vi "errorToString.vi"(1 "error in":errorcluster) -> (0 "Error Message":string)   [LabVIEW 2021]
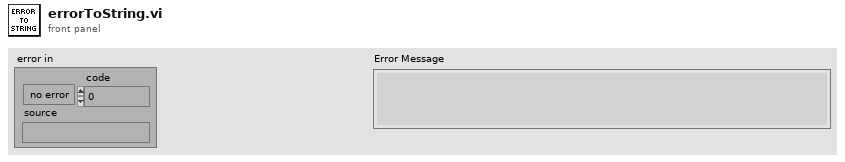
[diagram p1: front panel]
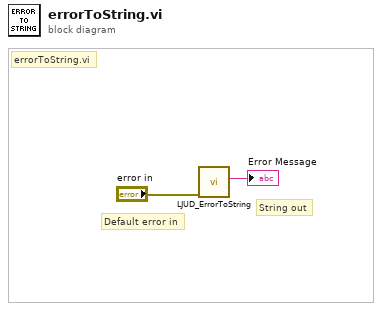
[diagram p0: block diagram]
diagram:
  # "errorToString.vi"
  # "String out"
  # "Default error in"
  n1 = call <vilib>:"LJUD_ErrorToString.vi"("error in"="error in") -> ("String"=→"Error Message":string)  [unwired: 10 in]
